vi "異常履歷.vi"() -> ()   [LabVIEW 2015]
panel:
  in  "²§±`¼i¾ú_§R°£":bool
  in  "Tab Control":enum32{"即時", "歷史紀錄"}(tab)
  in  "歷史訊息":bool caption="異常履歷_讀取"
  in  "即時現況":bool caption="異常履歷_讀取"
  in  "異常檔案":u16(ring) items=["2017¦~01¤ë06¤é.txt", "2017¦~01¤ë05¤é.txt", "2017¦~01¤ë04¤é.txt", "2017¦~01¤ë03¤é.txt", "2016¦~12¤ë29¤é.txt", "2016¦~12¤ë28¤é.txt", "2016¦~12¤ë27¤é.txt", "2016¦~12¤ë26¤é.txt", "2016¦~12¤ë25¤é.txt", "2016¦~12¤ë24¤é.txt", "2016¦~12¤ë23¤é.txt", "2016¦~12¤ë22¤é.txt", "2016¦~12¤ë21¤é.txt", "2016¦~12¤ë20¤é.txt", "2016¦~12¤ë19¤é.txt", "2016¦~12¤ë18¤é.txt", "2016¦~12¤ë17¤é.txt", "2016¦~12¤ë16¤é.txt", "2016¦~12¤ë14¤é.txt", "2016¦~12¤ë13¤é.txt", "2016¦~12¤ë12¤é.txt", "2016¦~12¤ë11¤é.txt", "2016¦~12¤ë10¤é.txt", "2016¦~12¤ë09¤é.txt", "2016¦~12¤ë08¤é.txt", "2016¦~12¤ë07¤é.txt", "2016¦~12¤ë06¤é.txt", "2016¦~12¤ë05¤é.txt", "2016¦~12¤ë04¤é.txt", "2016¦~12¤ë03¤é.txt", "2016¦~12¤ë02¤é.txt", "2016¦~12¤ë01¤é.txt", "2016¦~11¤ë30¤é.txt", "2016¦~11¤ë29¤é.txt", "2016¦~11¤ë28¤é.txt", "2016¦~11¤ë27¤é.txt", "2016¦~11¤ë26¤é.txt", "2016¦~11¤ë25¤é.txt", "2016¦~11¤ë24¤é.txt", "2016¦~11¤ë23¤é.txt", "2016¦~11¤ë22¤é.txt", "2016¦~11¤ë21¤é.txt", "2016¦~11¤ë20¤é.txt", "2016¦~11¤ë19¤é.txt", "2016¦~11¤ë18¤é.txt", "2016¦~11¤ë17¤é.txt", "2016¦~11¤ë16¤é.txt", "2016¦~11¤ë15¤é.txt", "2016¦~11¤ë14¤é.txt", "2016¦~11¤ë13¤é.txt", "2016¦~11¤ë12¤é.txt", "2016¦~11¤ë11¤é.txt"]
  in  "異常履歷_讀取":bool
  out "異常履歷":string[][](table)
  in  "Exit":bool
  # "Error Message"
  # "即時現況"
  # "歷史訊息"
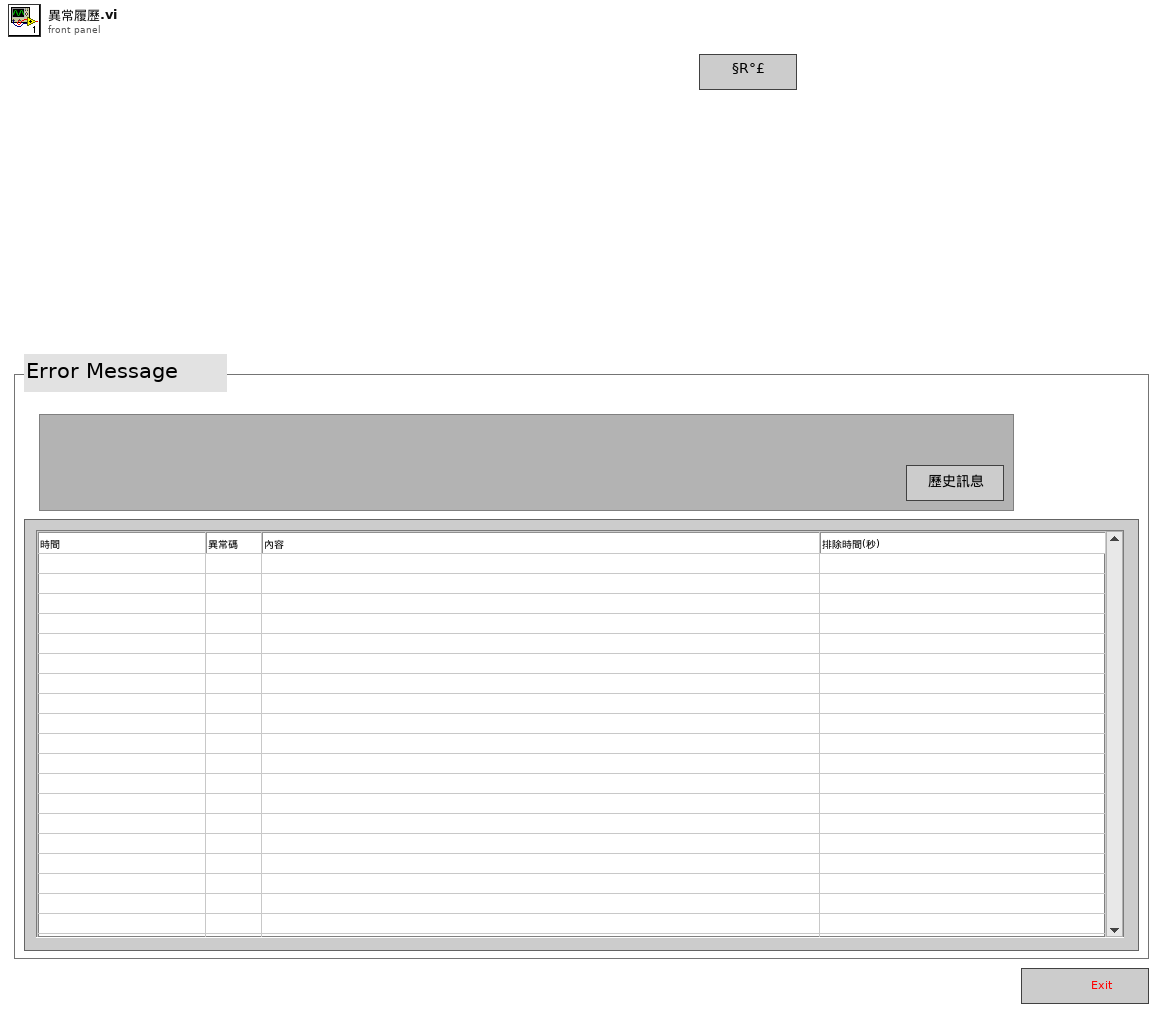
[diagram p1: front panel]
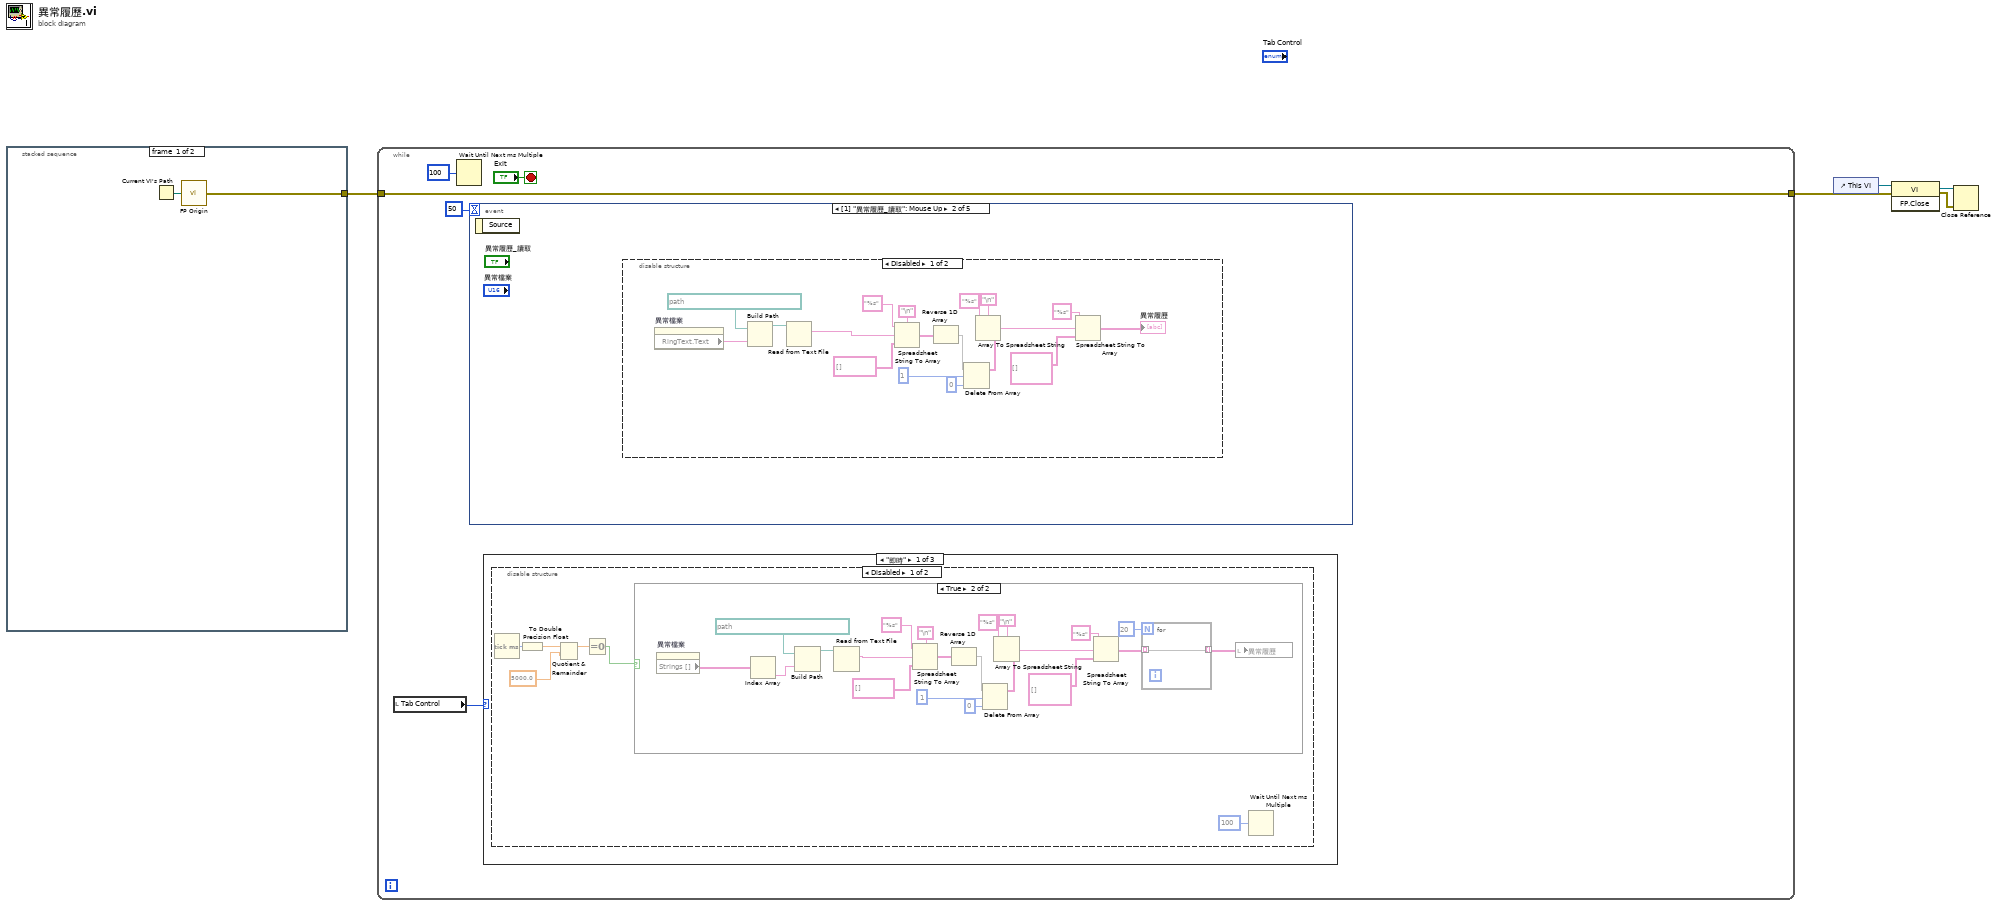
[diagram p0: block diagram]
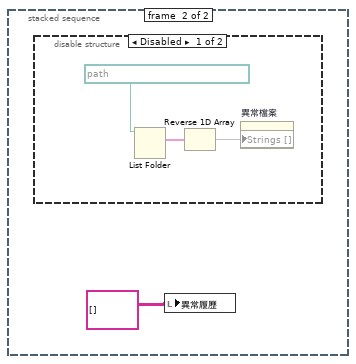
[diagram p2: hidden frame]
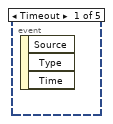
[diagram p8: hidden frame]
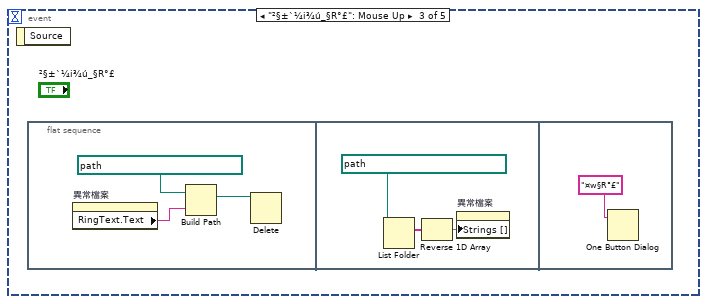
[diagram p10: hidden frame]
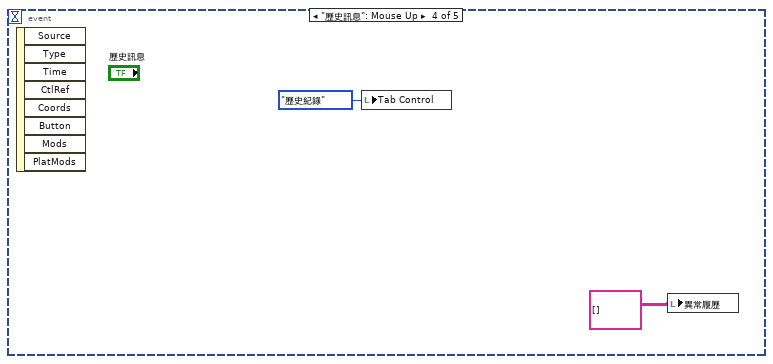
[diagram p11: hidden frame]
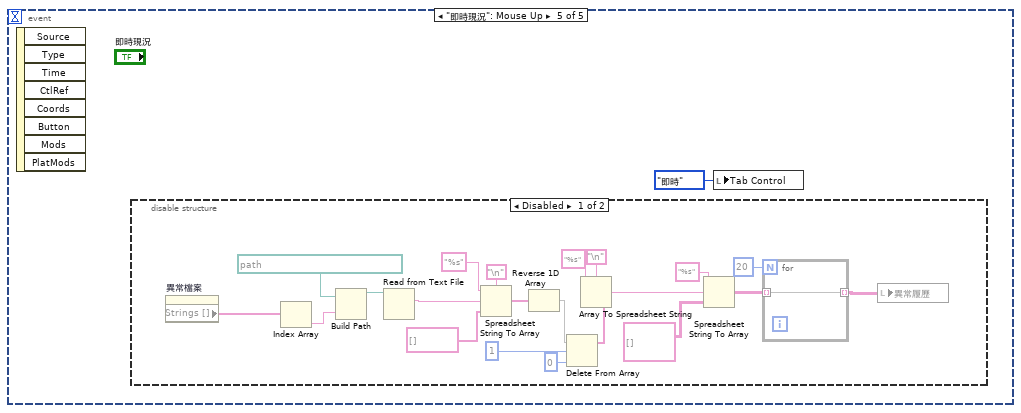
[diagram p12: hidden frame]
diagram:
  n1 = stacked-sequence {
    tunnel: [w6 _] -> w4
    frame #0 {
      n2 = Current VI's Path() -> (path=w7:path)
      n3 = call "FP Origin.vi"("vi path"=w7) -> ("error out"=w6:errorcluster)
    }
    frame #1 {
      n4 = disable-structure shown="Disabled" {
        frame Disabled {
          n5 = List Folder(path=path "D:/半自動電檢機 Data/Error" ("configuration file path")) -> (filenames=w10:string[])  [unwired: 3 in, 3 out]
          n6 = Reverse 1D Array(array=w10) -> (reversed array=w9:string[])
          n7 = property on="異常檔案" class="Ring (strict)"("Strings []"=w9) -> ()  [unwired: 2 in, 2 out]
        }
        frame Enabled {
        }
      }
      n8 = local write "異常履歷"(string[][] [] ("History")) -> ()
    }
  }
  n9 = while {
    tunnel: w4 -> [w13]
    tunnel: [w13] -> w5
    stop <- "Exit" stop-if-true
    n10 = local read "Tab Control"() -> (w12:enum32{"即時", "歷史紀錄"})
    n11 = Wait Until Next ms Multiple(millisecond multiple=u32 100) -> ()  [unwired: 1 out]
    n12 = event shown="[1] \"異常履歷_讀取\": Mouse Up" {
      selector: _ -> [_ _ _ _ _]
      dyn-events: _ -> [_ _ _ _ _]
      timeout: 50 -> [_ _ _ _ _]
      event Timeout {
        n13 = event-data() -> ()  [unwired: 1 in, 3 out]
      }
      event "異常履歷_讀取": Mouse Up {
        n14 = event-data() -> ()  [unwired: 1 in, 1 out]
        n15 = disable-structure shown="Disabled" {
          frame Disabled {
            n16 = property on="異常檔案" class="Ring (strict)"() -> ("RingText.Text"=w61:string)  [unwired: 2 in, 2 out]
            n17 = Build Path(base path=path "D:/半自動電檢機 Data/Error" ("configuration file path"), name or relative path=w61) -> (appended path=w62:path)
            n18 = Read from Text File(file (use dialog)=w62) -> (text=w45:string)  [unwired: 3 in, 3 out]
            n19 = Spreadsheet String To Array(delimiter (Tab)="\n", format string="%s", spreadsheet string=w45, array type (2D Dbl)=string[] []) -> (array=w53:string[])
            n20 = Reverse 1D Array(array=w53) -> (reversed array=w52:string[])
            n21 = Delete From Array(array=w52, length=1, index=0) -> (array with subset deleted=w49:string[])  [unwired: 1 out]
            n22 = Array To Spreadsheet String(delimiter (Tab)="\n", array=w49, 3:"%s" ("format string")) -> (spreadsheet string=w56:string)
            n23 = Spreadsheet String To Array(format string="%s", spreadsheet string=w56, array type (2D Dbl)=string[][] [] ("History")) -> (array=→"異常履歷":string[][])  [unwired: 1 in]
          }
          frame Enabled {
          }
        }
      }
      event "²§±`¼i¾ú_§R°£": Mouse Up {
        n24 = event-data() -> ()  [unwired: 1 in, 1 out]
        n25 = flat-sequence {
          frame #0 {
            n26 = property on="異常檔案" class="Ring (strict)"() -> ("RingText.Text"=w64:string)  [unwired: 2 in, 2 out]
            n27 = Build Path(base path=path "D:/半自動電檢機 Data/Error" ("configuration file path"), name or relative path=w64) -> (appended path=w65:path)
            n28 = Delete(path (use dialog)=w65) -> ()  [unwired: 4 in, 3 out]
          }
          frame #1 {
            n29 = List Folder(path=path "D:/半自動電檢機 Data/Error" ("configuration file path")) -> (filenames=w67:string[])  [unwired: 3 in, 3 out]
            n30 = Reverse 1D Array(array=w67) -> (reversed array=w66:string[])
            n31 = property on="異常檔案" class="Ring (strict)"("Strings []"=w66) -> ()  [unwired: 2 in, 2 out]
          }
          frame #2 {
            n32 = One Button Dialog(message="¤w§R°£") -> ()  [unwired: 1 in, 1 out]
          }
        }
      }
      event "歷史訊息": Mouse Up {
        n33 = event-data() -> ()  [unwired: 1 in, 8 out]
        n34 = local write "Tab Control"(enum32{"即時", "歷史紀錄"}."歷史紀錄" ("Tab Control")) -> ()
        n35 = local write "異常履歷"(string[][] [] ("History")) -> ()
      }
      event "即時現況": Mouse Up {
        n36 = event-data() -> ()  [unwired: 1 in, 8 out]
        n37 = disable-structure shown="Disabled" {
          frame Disabled {
            n38 = property on="異常檔案" class="Ring (strict)"() -> ("Strings []"=w88:string[])  [unwired: 2 in, 2 out]
            n39 = Index Array(array=w88) -> (element=w89:string)  [unwired: 1 in]
            n40 = Build Path(base path=path "D:/半自動電檢機 Data/Error" ("configuration file path"), name or relative path=w89) -> (appended path=w93:path)
            n41 = Read from Text File(file (use dialog)=w93) -> (text=w84:string)  [unwired: 3 in, 3 out]
            n42 = Spreadsheet String To Array(delimiter (Tab)="\n", format string="%s", spreadsheet string=w84, array type (2D Dbl)=string[] []) -> (array=w79:string[])
            n43 = Reverse 1D Array(array=w79) -> (reversed array=w78:string[])
            n44 = Delete From Array(array=w78, length=1, index=0) -> (array with subset deleted=w75:string[])  [unwired: 1 out]
            n45 = Array To Spreadsheet String(delimiter (Tab)="\n", array=w75, 3:"%s" ("format string")) -> (spreadsheet string=w82:string)
            n46 = Spreadsheet String To Array(format string="%s", spreadsheet string=w82, array type (2D Dbl)=string[][] [] ("History")) -> (array=w85:string[][])  [unwired: 1 in]
            n47 = for {
              N: 20 -> [_]
              tunnel: [w94] -> w86 mode=indexing
              tunnel: w85 -> [w94] mode=indexing
            }
            n48 = local write "異常履歷"(w86) -> ()
          }
          frame Enabled {
          }
        }
        n49 = local write "Tab Control"(enum32{"即時", "歷史紀錄"}."即時" ("Tab Control")) -> ()
      }
    }
    n50 = case shown="\"即時\"" w12 {
      frame "即時" {
        n51 = disable-structure shown="Disabled" {
          frame Disabled {
            n52 = Tick Count (ms)() -> (millisecond timer value=w21:u32)
            n53 = To Double Precision Float(number=w21) -> (double precision float=w20:dbl)
            n54 = Quotient & Remainder(x=w20, y=5000.0) -> (x-y*floor(x/y)=w18:dbl)  [unwired: 1 out]
            n55 = Equal To 0?(x=w18) -> (x = 0?=w17:bool)
            n56 = case shown="True" w17 {
              frame False {
              }
              frame True {
                n57 = property on="異常檔案" class="Ring (strict)"() -> ("Strings []"=w28:string[])  [unwired: 2 in, 2 out]
                n58 = Index Array(array=w28) -> (element=w27:string)  [unwired: 1 in]
                n59 = Build Path(base path=path "D:/半自動電檢機 Data/Error" ("configuration file path"), name or relative path=w27) -> (appended path=w23:path)
                n60 = Read from Text File(file (use dialog)=w23) -> (text=w32:string)  [unwired: 3 in, 3 out]
                n61 = Spreadsheet String To Array(delimiter (Tab)="\n", format string="%s", spreadsheet string=w32, array type (2D Dbl)=string[] []) -> (array=w37:string[])
                n62 = Reverse 1D Array(array=w37) -> (reversed array=w38:string[])
                n63 = Delete From Array(array=w38, length=1, index=0) -> (array with subset deleted=w41:string[])  [unwired: 1 out]
                n64 = Array To Spreadsheet String(delimiter (Tab)="\n", array=w41, 3:"%s" ("format string")) -> (spreadsheet string=w34:string)
                n65 = Spreadsheet String To Array(format string="%s", spreadsheet string=w34, array type (2D Dbl)=string[][] [] ("History")) -> (array=w31:string[][])  [unwired: 1 in]
                n66 = for {
                  N: 20 -> [_]
                  tunnel: [w44] -> w30 mode=indexing
                  tunnel: w31 -> [w44] mode=indexing
                }
                n67 = local write "異常履歷"(w30) -> ()
              }
            }
            n68 = Wait Until Next ms Multiple(millisecond multiple=u32 100) -> ()  [unwired: 1 out]
          }
          frame Enabled {
          }
        }
      }
      frame Default {
      }
      frame "歷史紀錄" {
      }
    }
  }
  n69 = control-ref of="This VI"() -> (w3:refnum<vi>)
  n70 = invoke class="VI" method="FP.Close"(reference=w3, error in=w5) -> (reference out=w2:refnum<vi>, error out=w1:errorcluster)  [unwired: 1 in, 1 out]
  n71 = Close Reference(reference=w2, error in (no error)=w1) -> ()  [unwired: 1 out]
